vi "Search for sequence.vi"(10 "Pattern For Number Of Letters":string, 11 "Array":string[][](array[string])) -> (3 "sequence":string)   [LabVIEW 2019, in "Day 8.lvlib"]
uses:
  Day 8.lvlib
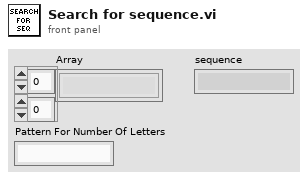
[diagram p1: front panel]
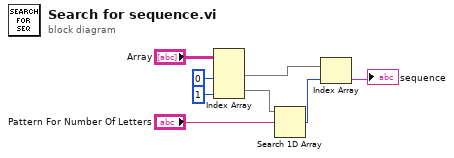
[diagram p0: block diagram]
diagram:
  n1 = Index Array(array="Array", index (col) #1=0 ("disabled index (col)"), index (col) #2=1 ("disabled index (col)")) -> (element #1=w5:string[], element #2=w7:string[])  [unwired: 2 in]
  n2 = Search 1D Array(1D array=w7, element="Pattern For Number Of Letters") -> (index of element=w6:i32)  [unwired: 1 in]
  n3 = Index Array(array=w5, index=w6) -> (element=→"sequence":string)
